vi "SaveImage.vi"(7 "Path":path, 8 "EN":bool, 9 "Test Name":string, 10 "XYG_Up":refnum<vi>, 11 "XYG_Down":refnum<vi>) -> ()   [LabVIEW 2017]
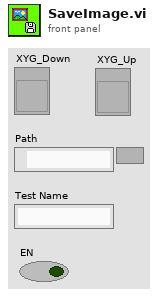
[diagram p1: front panel]
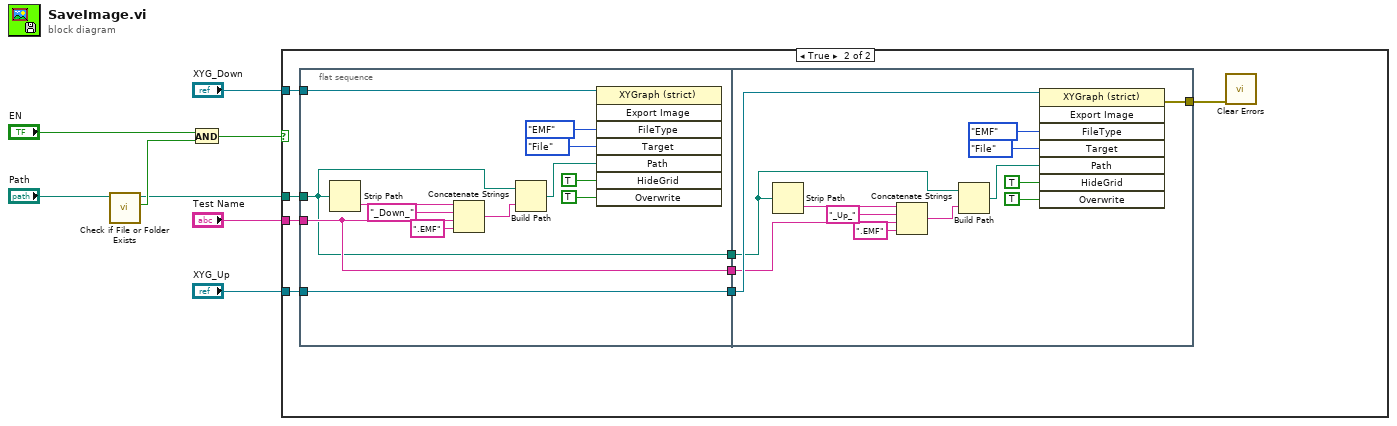
[diagram p0: block diagram]
diagram:
  n1 = call <vilib>:"Check if File or Folder Exists.vi"("path"="Path") -> ("file or folder exists?"=w3:bool, "dup path"=w2:path)  [unwired: 8 in, 1 out]
  n2 = And(x="EN", y=w3) -> (x .and. y?=w5:bool)
  n3 = case shown="True" w5 {
    tunnel: "XYG_Down" -> [_ w16]
    tunnel: "Test Name" -> [_ w15]
    tunnel: w2 -> [_ w14]
    tunnel: "XYG_Up" -> [_ w12]
    frame False {
    }
    frame True {
      n4 = flat-sequence {
        tunnel: w16 -> [w29]
        tunnel: w15 -> [w18]
        tunnel: w14 -> [w17]
        tunnel: [w19] -> w13
        tunnel: w12 -> [w19]
        tunnel: [w18] -> w11
        tunnel: [w17] -> w10
        tunnel: w13 -> [w33]
        tunnel: w11 -> [w32]
        tunnel: w10 -> [w31]
        tunnel: [w30] -> w9
        frame #0 {
          n5 = Strip Path(path=w17) -> (name=w24:string)  [unwired: 1 out]
          n6 = Concatenate Strings(w24, "_Down_" ("string"), w18, ".EMF" ("string")) -> (w21:string)
          n7 = Build Path(base path=w17, name or relative path=w21) -> (appended path=w20:path)
          n8 = invoke class="XYGraph (strict)" method="Export Image"(reference=w29, "FileType"=enum32{"BMP", "EPS", "EMF", "PICT"}."EMF" ("File Type"), "Target"=enum32{"File", "Clipboard"}."File", "Path"=w20, "HideGrid"=TRUE ("Hide Grid"), "Overwrite"=TRUE ("Always Overwrite")) -> ()  [unwired: 2 in, 8 out]
        }
        frame #1 {
          n9 = Strip Path(path=w31) -> (name=w38:string)  [unwired: 1 out]
          n10 = Concatenate Strings(w38, "_Up_" ("string"), w32, ".EMF" ("string")) -> (w41:string)
          n11 = Build Path(base path=w31, name or relative path=w41) -> (appended path=w42:path)
          n12 = invoke class="XYGraph (strict)" method="Export Image"(reference=w33, "FileType"=enum32{"BMP", "EPS", "EMF", "PICT"}."EMF" ("File Type"), "Target"=enum32{"File", "Clipboard"}."File", "Path"=w42, "HideGrid"=TRUE ("Hide Grid"), "Overwrite"=TRUE ("Always Overwrite")) -> (error out=w30:errorcluster)  [unwired: 2 in, 7 out]
        }
      }
      n13 = call <vilib>:"Clear Errors.vi"("error in (no error)"=w9) -> ()  [unwired: 5 in, 2 out]
    }
  }
